vi "Arm_LE_To_XZ.vi"(9 "Extend":dbl, 10 "Lift":dbl) -> (1 "z":dbl, 3 "x":dbl)   [LabVIEW 2020]
uses:
  <vilib>/Rock Robotics/WPI/ThirdParty/JAS_Junk/TrajLib/Trajectory_Library.lvlib
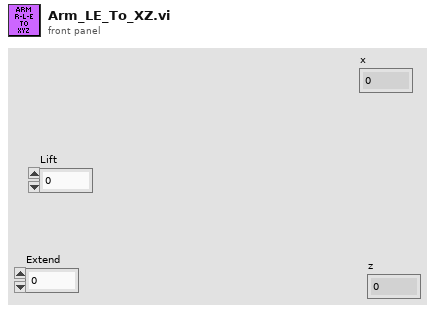
[diagram p1: front panel]
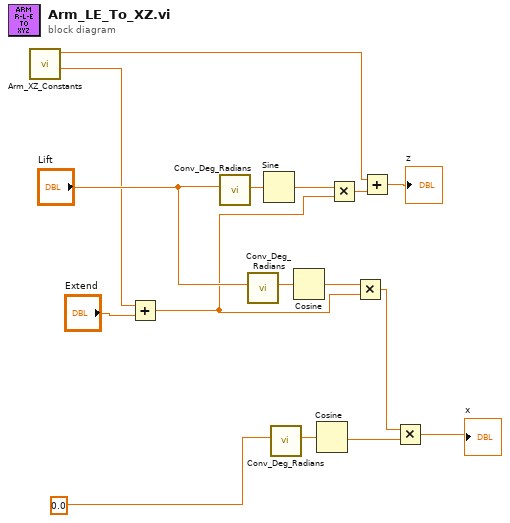
[diagram p0: block diagram]
diagram:
  n1 = call "Arm_XZ_Constants.vi"() -> ("Unextended Length (in)"=w2:dbl, "Pivot Height (in)"=w3:dbl)  [unwired: 10 in]
  n2 = Add(x=w2, y="Extend") -> (x+y=w10:dbl)
  n3 = call <vilib>:"Conv_Deg_Radians.vi"("Degress"="Lift") -> ("Radians"=w16:dbl)  [unwired: 10 in]
  n4 = call <vilib>:"Conv_Deg_Radians.vi"("Degress"="Lift") -> ("Radians"=w13:dbl)  [unwired: 10 in]
  n5 = Sine(x=w16) -> (sin(x)=w14:dbl)
  n6 = call <vilib>:"Conv_Deg_Radians.vi"("Degress"=0.0) -> ("Radians"=w9:dbl)  [unwired: 10 in]
  n7 = Cosine(x=w13) -> (cos(x)=w11:dbl)
  n8 = Cosine(x=w9) -> (cos(x)=w8:dbl)
  n9 = Multiply(x=w14, y=w10) -> (x*y=w5:dbl)
  n10 = Multiply(x=w11, y=w10) -> (x*y=w6:dbl)
  n11 = Add(x=w3, y=w5) -> (x+y=→"z":dbl)
  n12 = Multiply(x=w6, y=w8) -> (x*y=→"x":dbl)
